vi "main.vi"() -> ()   [LabVIEW 2018]
uses:
  <vilib>/Utility/config.llb/Write Key (Double).vi
  <vilib>/Utility/config.llb/Write Key (U32).vi
  <vilib>/Utility/config.llb/Write Key (Boolean).vi
  <vilib>/Utility/config.llb/Write Key (I32).vi
  <vilib>/Utility/config.llb/NI_LVConfig.lvlib
panel:
  in  "脉冲开关 2":bool
  in  "选项卡控件":enum32{"Graph", "All channel", "Single channel"}(tab)
  out "波形图表时间簇1":cluster{"起始":dbl, "中间":dbl, "终止":dbl}={"起始"=0.0, "中间"=2.5, "终止"=5.0} {"起始" format="%#.1p"; "终止" format="%#.1p"; "中间" format="%#.1p"}
  out "Chart1":waveform(dbl)[](graph)
  out "波形图表时间簇2":cluster{"起始":dbl, "中间":dbl, "终止":dbl}={"起始"=0.0, "中间"=2.5, "终止"=5.0} {"起始" format="%#.1p"; "终止" format="%#.1p"; "中间" format="%#.1p"}
  out "Chart2":waveform(dbl)[](graph)
  out "波形图表时间簇3":cluster{"起始":dbl, "中间":dbl, "终止":dbl}={"起始"=0.0, "中间"=2.5, "终止"=5.0} {"起始" format="%#.1p"; "终止" format="%#.1p"; "中间" format="%#.1p"}
  out "Chart3":waveform(dbl)[](graph)
  out "波形图表时间簇4":cluster{"起始":dbl, "中间":dbl, "终止":dbl}={"起始"=0.0, "中间"=2.5, "终止"=5.0} {"起始" format="%#.1p"; "终止" format="%#.1p"; "中间" format="%#.1p"}
  out "Chart4":waveform(dbl)[](graph)
  in  "全部":T1={"Amp"=1.0, "Fre"=2, "Wid"=20, "选通"=TRUE, "脉宽单位"=enum."us", "字符串"="全部", "Time"=2} {"Wid" min=1 step=1; "Amp" min=0 max=15 step=0.1 format="%#_3f"}
  in  "所有保存配置":bool
  out "Path":path
  in  "单独保存配置":bool
  in  "读取配置":bool
  in  "Configuration select":path
  out "Configuration save":path
  in  "Information":T2(array[cluster])=[[{"Amp"=10.0, "Fre"=1, "Wid"=200, "选通"=TRUE, "脉宽单位"=enum."us", "字符串"="CH0", "Time"=1}, {"Amp"=2.0, "Fre"=2, "Wid"=200, "选通"=FALSE, "脉宽单位"=enum."us", "字符串"="CH1", "Time"=2}, {"Amp"=1.0, "Fre"=3, "Wid"=200, "选通"=FALSE, "脉宽单位"=enum."us", "字符串"="CH2", "Time"=3}, {"Amp"=1.0, "Fre"=4, "Wid"=200, "选通"=FALSE, "脉宽单位"=enum."us", "字符串"="CH3", "Time"=4}, {"Amp"=2.0, "Fre"=5, "Wid"=200, "选通"=FALSE, "脉宽单位"=enum."us", "字符串"="CH4", "Time"=5}, {"Amp"=3.0, "Fre"=6, "Wid"=200, "选通"=FALSE, "脉宽单位"=enum."us", "字符串"="CH5", "Time"=6}, {"Amp"=2.0, "Fre"=7, "Wid"=200, "选通"=FALSE, "脉宽单位"=enum."us", "字符串"="CH6", "Time"=7}, {"Amp"=10.0, "Fre"=8, "Wid"=200, "选通"=FALSE, "脉宽单位"=enum."us", "字符串"="CH7", "Time"=8}], [{"Amp"=1.0, "Fre"=1, "Wid"=200, "选通"=FALSE, "脉宽单位"=enum."us", "字符串"="CH8", "Time"=9}, {"Amp"=1.0, "Fre"=2, "Wid"=200, "选通"=FALSE, "脉宽单位"=enum."us", "字符串"="CH9", "Time"=10}, {"Amp"=1.0, "Fre"=3, "Wid"=200, "选通"=FALSE, "脉宽单位"=enum."us", "字符串"="CH10", "Time"=11}, {"Amp"=1.0, "Fre"=4, "Wid"=200, "选通"=FALSE, "脉宽单位"=enum."us", "字符串"="CH11", "Time"=12}, {"Amp"=1.0, "Fre"=5, "Wid"=200, "选通"=TRUE, "脉宽单位"=enum."us", "字符串"="CH12", "Time"=13}, {"Amp"=1.0, "Fre"=6, "Wid"=200, "选通"=FALSE, "脉宽单位"=enum."us", "字符串"="CH13", "Time"=14}, {"Amp"=1.0, "Fre"=7, "Wid"=200, "选通"=FALSE, "脉宽单位"=enum."us", "字符串"="CH14", "Time"=15}, {"Amp"=1.0, "Fre"=8, "Wid"=200, "选通"=FALSE, "脉宽单位"=enum."us", "字符串"="CH15", "Time"=16}], [{"Amp"=1.0, "Fre"=1, "Wid"=200, "选通"=FALSE, "脉宽单位"=enum."us", "字符串"="CH16", "Time"=1}, {"Amp"=1.0, "Fre"=2, "Wid"=200, "选通"=FALSE, "脉宽单位"=enum."us", "字符串"="CH17", "Time"=2}, {"Amp"=1.0, "Fre"=3, "Wid"=200, "选通"=FALSE, "脉宽单位"=enum."us", "字符串"="CH18", "Time"=3}, {"Amp"=1.0, "Fre"=4, "Wid"=200, "选通"=TRUE, "脉宽单位"=enum."us", "字符串"="CH19", "Time"=4}, {"Amp"=1.0, "Fre"=5, "Wid"=200, "选通"=FALSE, "脉宽单位"=enum."us", "字符串"="CH20", "Time"=5}, {"Amp"=1.0, "Fre"=6, "Wid"=200, "选通"=TRUE, "脉宽单位"=enum."us", "字符串"="CH21", "Time"=6}, {"Amp"=1.0, "Fre"=7, "Wid"=200, "选通"=FALSE, "脉宽单位"=enum."us", "字符串"="CH22", "Time"=7}, {"Amp"=1.0, "Fre"=8, "Wid"=200, "选通"=FALSE, "脉宽单位"=enum."us", "字符串"="CH23", "Time"=8}], [{"Amp"=1.0, "Fre"=1, "Wid"=200, "选通"=FALSE, "脉宽单位"=enum."us", "字符串"="CH24", "Time"=1}, {"Amp"=1.0, "Fre"=2, "Wid"=200, "选通"=FALSE, "脉宽单位"=enum."us", "字符串"="CH25", "Time"=2}, {"Amp"=1.0, "Fre"=2, "Wid"=200, "选通"=FALSE, "脉宽单位"=enum."us", "字符串"="CH26", "Time"=3}, {"Amp"=1.0, "Fre"=2, "Wid"=200, "选通"=FALSE, "脉宽单位"=enum."us", "字符串"="CH27", "Time"=4}, {"Amp"=1.0, "Fre"=2, "Wid"=200, "选通"=FALSE, "脉宽单位"=enum."us", "字符串"="CH28", "Time"=5}, {"Amp"=1.0, "Fre"=31, "Wid"=200, "选通"=FALSE, "脉宽单位"=enum."us", "字符串"="CH29", "Time"=6}, {"Amp"=1.0, "Fre"=31, "Wid"=200, "选通"=FALSE, "脉宽单位"=enum."us", "字符串"="CH30", "Time"=7}, {"Amp"=1.0, "Fre"=31, "Wid"=200, "选通"=TRUE, "脉宽单位"=enum."us", "字符串"="CH31", "Time"=8}]] {"Wid" min=1 step=1; "Amp" min=0 max=15 step=0.1 format="%#_3f"}
  in  "Save path":path=path "C:/Users/86131/Desktop/新建文件夹"
  in  "打开TDMS":bool
  out "Record status":string
  in  "波形图表时间簇4 2":cluster{"起始":dbl, "中间":dbl, "终止":dbl} {"起始" format="%#.1p"; "终止" format="%#.1p"; "中间" format="%#.1p"}
  out "记录文件输出路径":path
  out "Countdown(s)":dbl format="%<%H:%M:%S>t"
  in  "Reocord mode":T3(ring)
  in  "Duration(s)":u32=10
  in  "Interval time(s)":i32=60 format="%<%H:%M:%S>t"
  in  "倒计时控制":bool
  out "tdms文件输出":refnum<k34>
  out "采集时间已到":bool
  in  "XScale":dbl(ring)=5.0 items=["10ms"=0.01, "100ms"=0.1, "1s"=1.0, "5s"=5.0, "10s"=10.0]
  in  "YScale":i16(ring)=5000 items=["+/-50μV"=50, "+/-100μV"=100, "+/-200μV"=200, "+/-500μV"=500, "+/-1mV"=1000, "+/-2mV"=2000, "+/-5mV"=5000, "+/-10mV"=10000]
  out "停止控制":bool=TRUE
  in  "停止按钮":bool
  in  "开始按钮":bool
  in  "记录开关":bool
  in  "脉冲开关":bool
  in  "命名方式":enum16{"电穿孔条件", "时间"}(ring)=enum."时间"
  # "Cell electrophysiological \nrecording system"
  # "Fixed time setting"
  # "CH0"
  # "CH1"
  # "CH2"
  # "CH3"
  # "CH4"
  # "CH5"
  # "CH6"
  # "CH7"
  # "CH8"
  # "CH9"
  # "CH10"
  # "CH11"
  # "CH12"
  # "CH13"
  # "CH14"
  # "CH15"
  # "CH16"
  # "CH17"
  # "CH18"
  # "CH19"
  # "CH20"
  # "CH21"
  # "CH22"
  # "CH23"
  # "CH24"
  # "CH25"
  # "CH26"
  # "CH27"
  # "CH28"
  # "CH29"
  # "CH30"
  # "CH31"
  # "V"
  # "Hz"
  # "s"
  # "V"
  # "Hz"
  # "s"
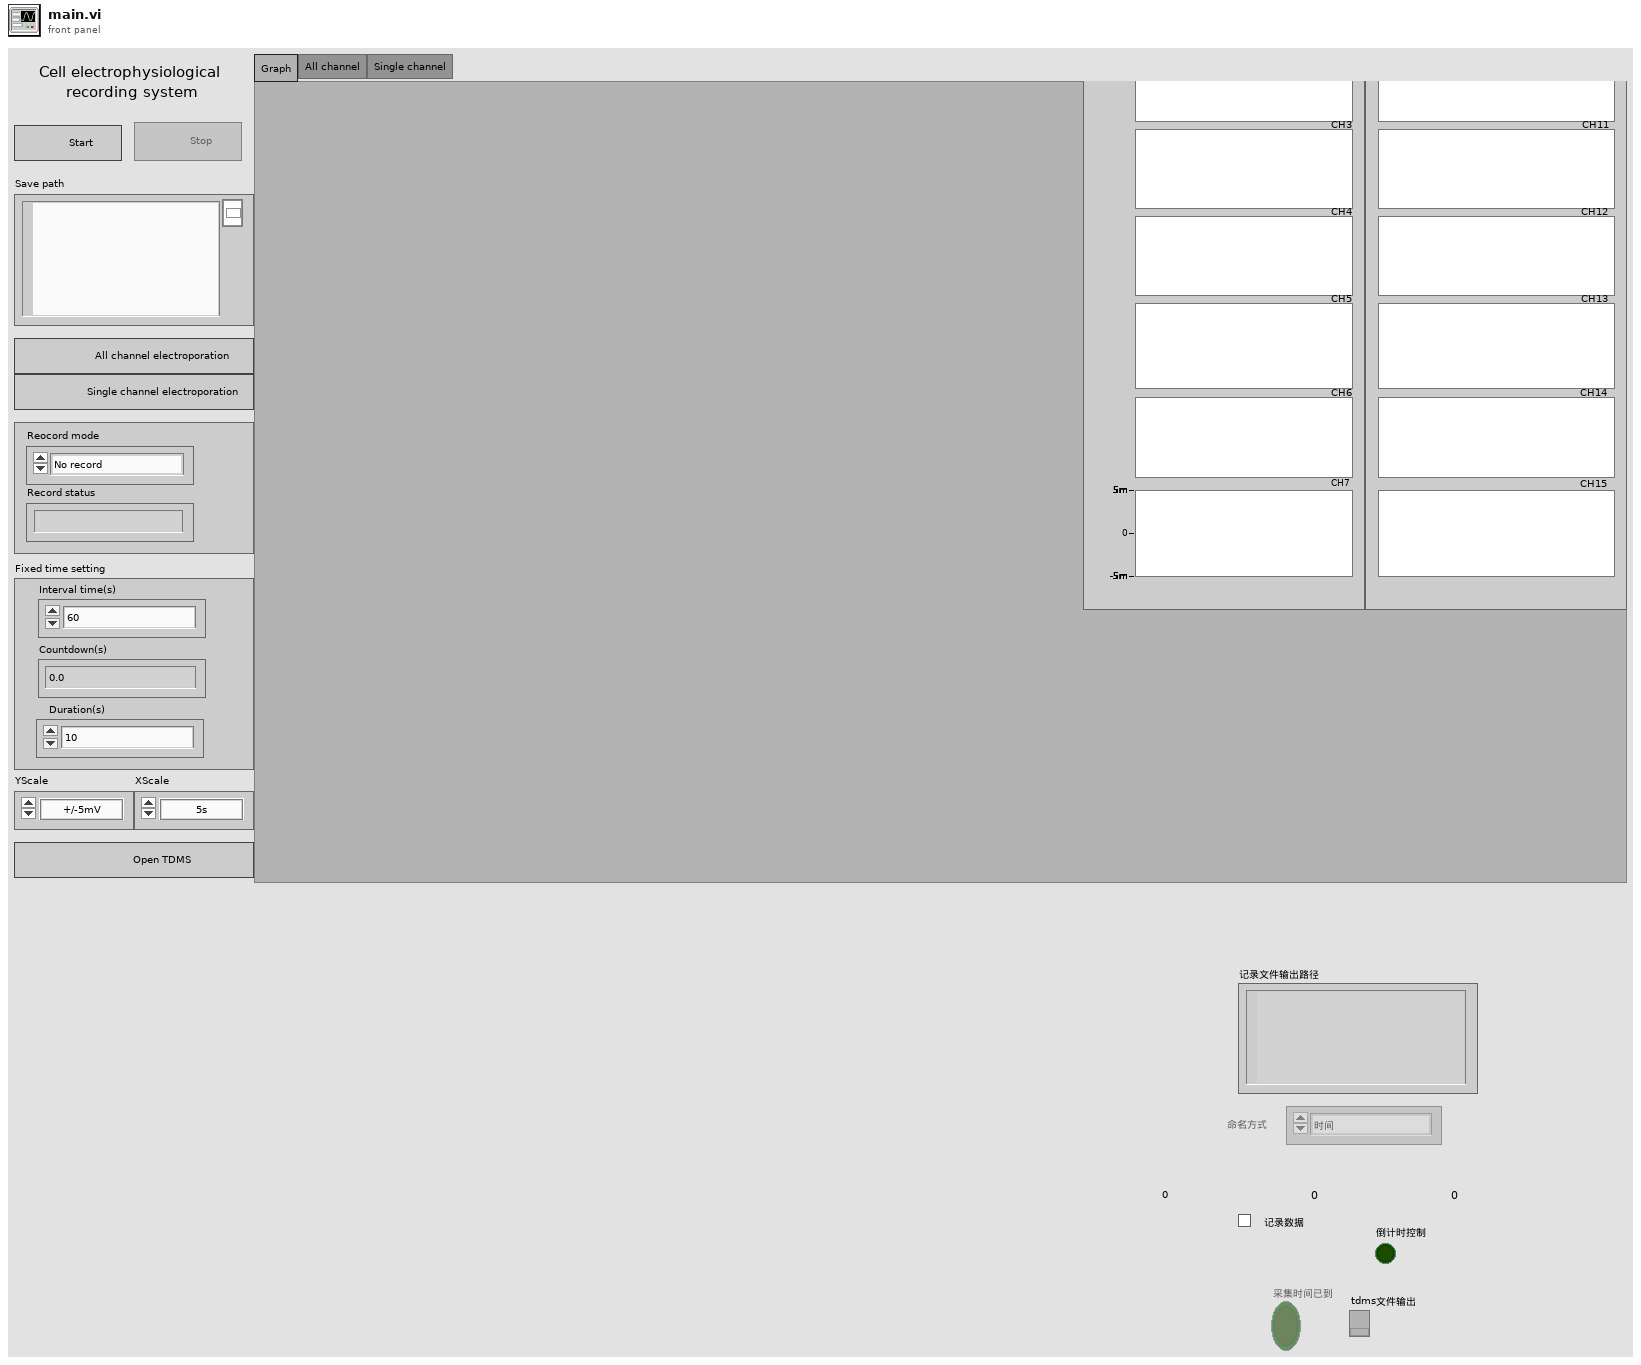
[diagram p1: front panel]
types:
  T1 = cluster{"Amp":sgl, "Fre":u32, "Wid":u16, "选通":bool, "脉宽单位":enum16{"ns", "us", "ms"}, "字符串":string, "Time":i32}
  T2 = cluster{"Amp":sgl, "Fre":u32, "Wid":u16, "选通":bool, "脉宽单位":enum16{"ns", "us", "ms"}, "字符串":string, "Time":i32}[][]
  T3 = enum16{"No record", "Continuous record", "Fixed time"}
  T4 = enum16{"open", "open or create", "create or replace", "create", "open (read-only)"}
  T5 = enum8{"Enabled", "Disabled", "Disabled and Grayed Out"}
  T6 = typedef "NI_LVConfig.lvlib/Config Data RefNum.ctl" = refnum<k1>
  T7 = cluster{"幅值":sgl, "频率":u32, "脉宽":u16, "选通":bool, "脉宽单位":enum16{"ns", "us", "ms"}, "字符串":string, "时间":i32}[][]
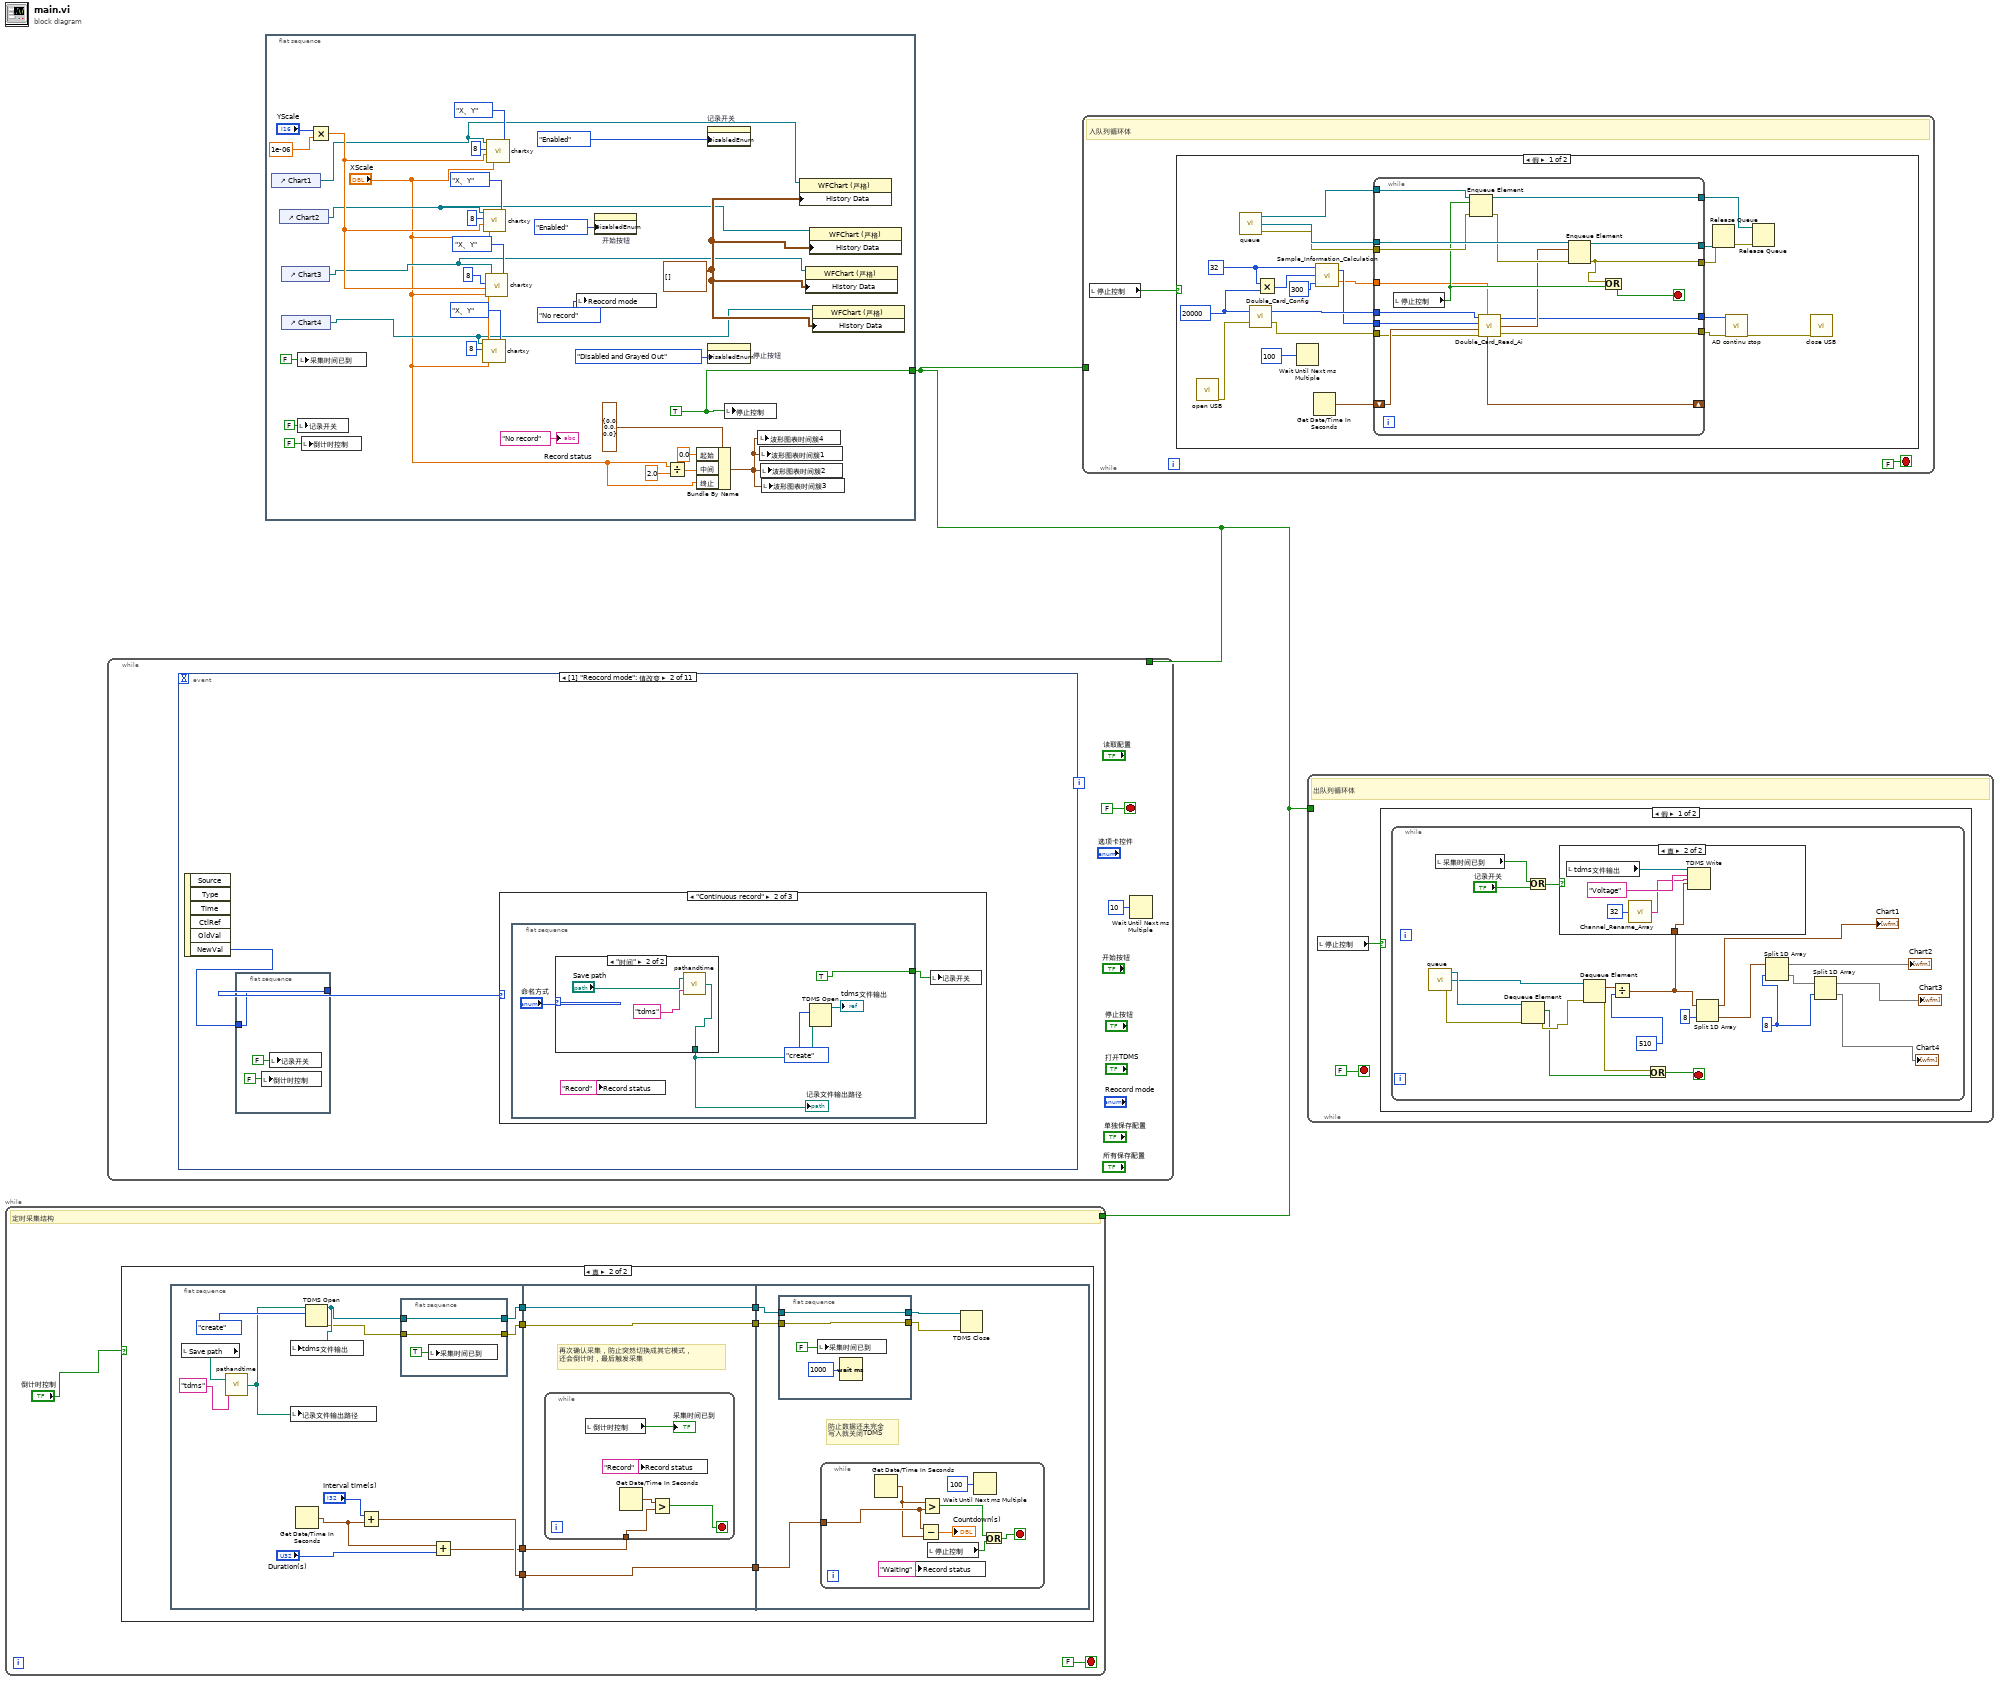
[diagram p0: block diagram]
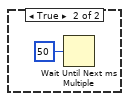
[diagram p3: hidden frame]
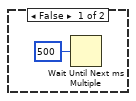
[diagram p4: hidden frame]
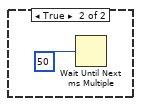
[diagram p5: hidden frame]
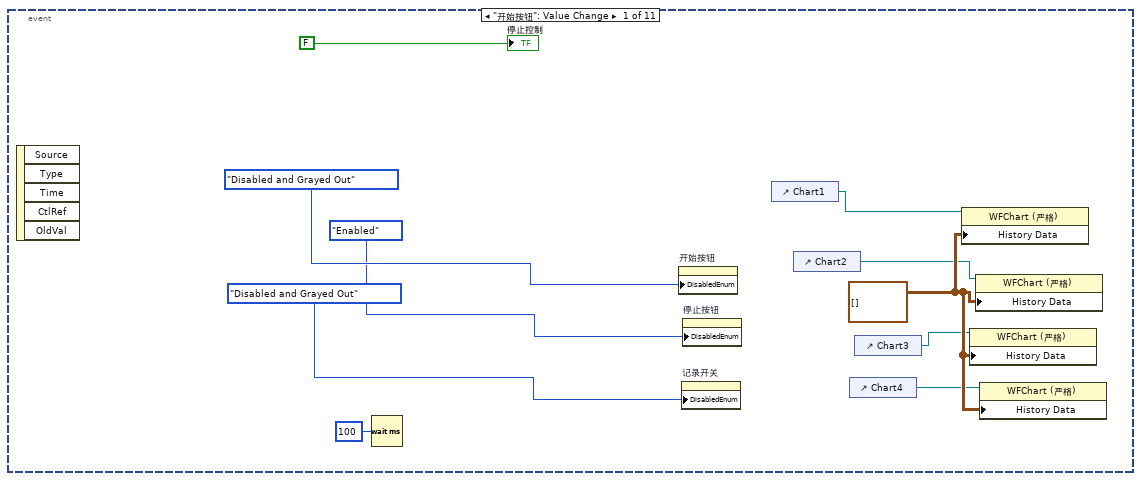
[diagram p6: hidden frame]
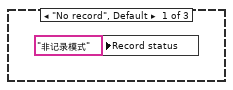
[diagram p7: hidden frame]
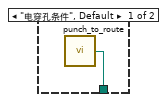
[diagram p8: hidden frame]
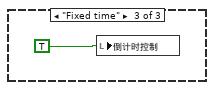
[diagram p9: hidden frame]
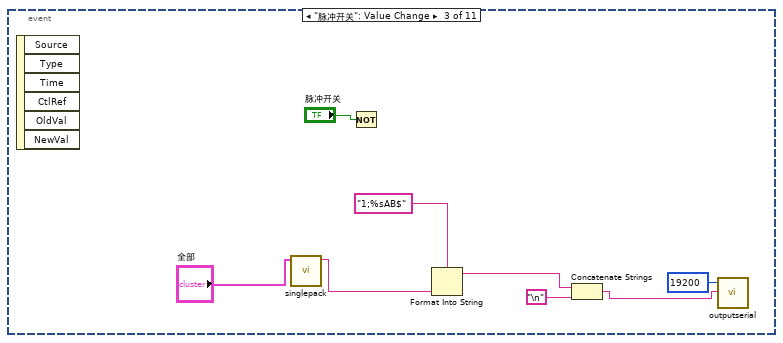
[diagram p10: hidden frame]
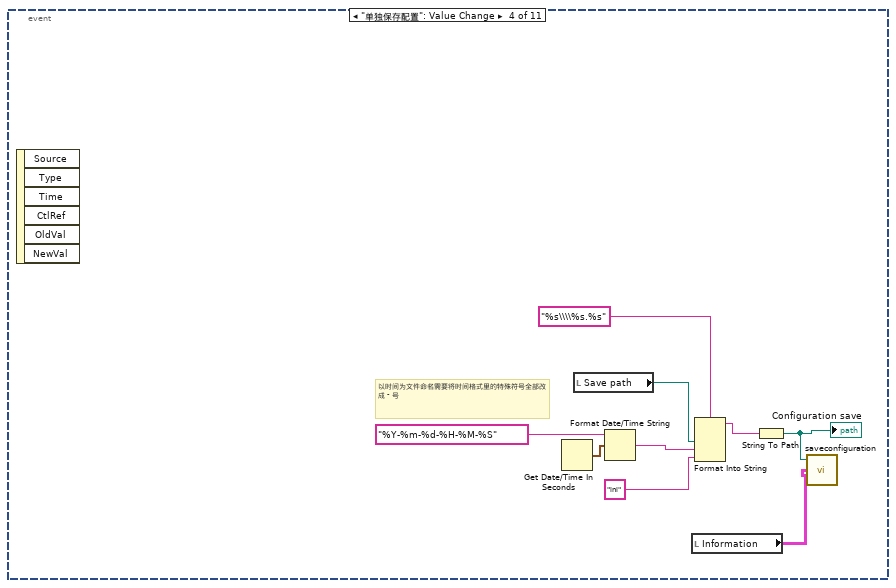
[diagram p11: hidden frame]
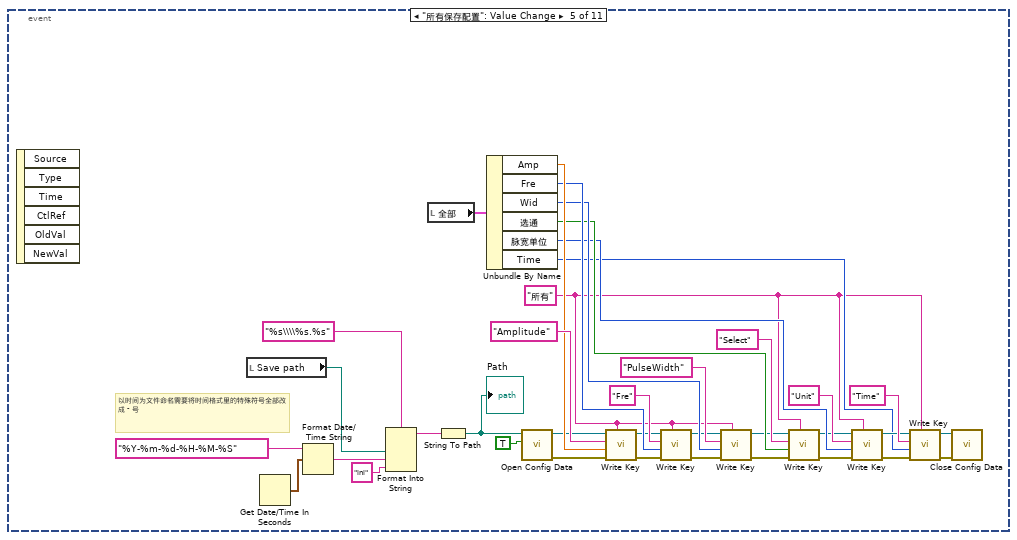
[diagram p12: hidden frame]
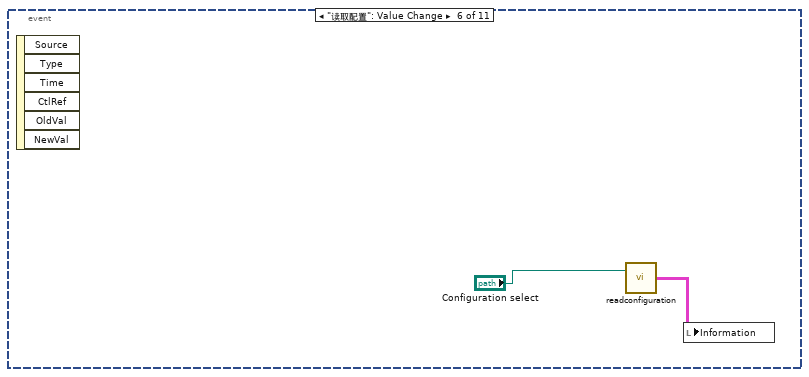
[diagram p13: hidden frame]
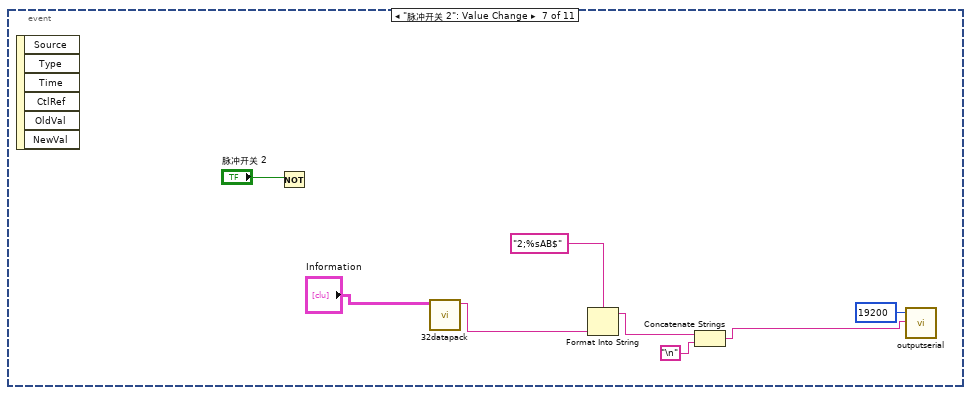
[diagram p14: hidden frame]
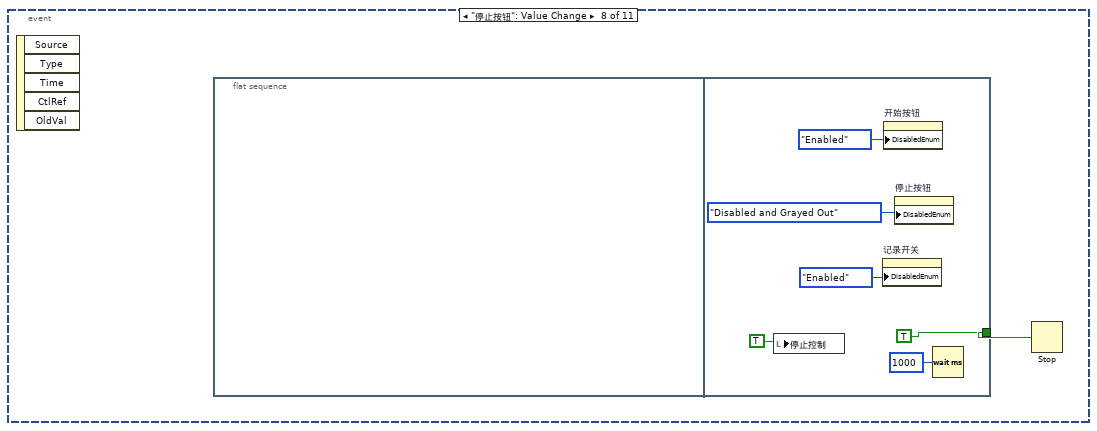
[diagram p15: hidden frame]
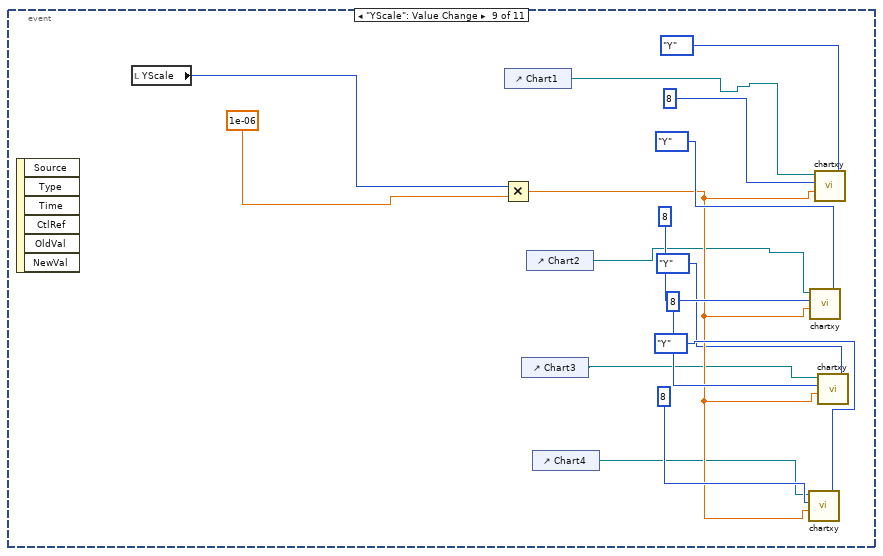
[diagram p16: hidden frame]
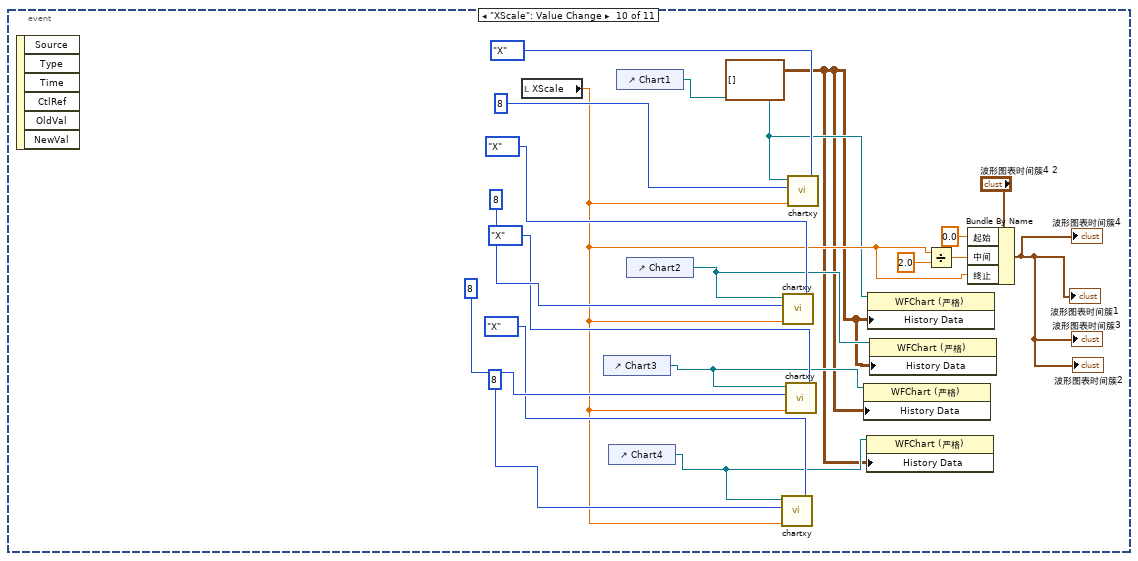
[diagram p17: hidden frame]
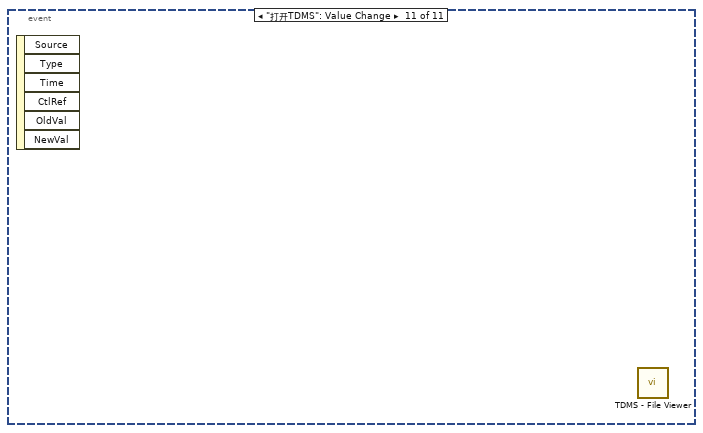
[diagram p18: hidden frame]
diagram:
  n1 = while {
    tunnel: w1 -> [_]
    stop <- FALSE stop-if-true
    # "定时采集结构"
    n2 = case shown="真" "倒计时控制" {
      frame False {
        n3 = Wait Until Next ms Multiple(millisecond multiple=u32 500 ("等待时间（毫秒）")) -> ()  [unwired: 1 out]
      }
      frame True {
        n4 = flat-sequence {
          tunnel: [w18] -> w11
          tunnel: [w16] -> w10
          tunnel: [w22] -> w6
          tunnel: [w19] -> w5
          tunnel: w11 -> [w31]
          tunnel: w10 -> [w30]
          tunnel: [w31] -> w9
          tunnel: [w30] -> w8
          tunnel: [w29] -> w7
          tunnel: w6 -> [w29]
          tunnel: w5 -> [w28]
          tunnel: w9 -> [w39]
          tunnel: w8 -> [w37]
          tunnel: w7 -> [w41]
          frame #0 {
            n5 = local read "Save path"() -> (w12:path)
            n6 = call "pathandtime.vi"("文件扩展名"="tdms", "文件路径输入控件"=w12) -> ("时间命名的文件路径"=w13:path)
            n7 = local write "记录文件输出路径"(w13) -> ()
            n8 = Get Date/Time In Seconds() -> (seconds since 1Jan1904=w20:timestamp)
            n9 = TDMS Open(10:T4."create" ("操作(0:open)"), 11:w13) -> (0:w15:errorcluster, 3:w17:refnum<k34>)  [unwired: 5 in]
            n10 = local write "tdms文件输出"(w17) -> ()
            n11 = Add(x="Interval time(s)", y=w20) -> (x+y=w22:timestamp)
            n12 = flat-sequence {
              tunnel: [w27] -> w18
              tunnel: w17 -> [w27]
              tunnel: [w26] -> w16
              tunnel: w15 -> [w26]
              frame #0 {
                n13 = local write "采集时间已到"(TRUE ("采集时间已到")) -> ()
              }
            }
            n14 = Add(x=w20, y="Duration(s)") -> (x+y=w19:timestamp)
          }
          frame #1 {
            # "再次确认采集，防止突然切换成其它模式，\n还会倒计时，最后触发采集"
            n15 = while {
              tunnel: w28 -> [w34]
              stop <- w33 stop-if-true
              n16 = local read "倒计时控制"() -> (→"采集时间已到":bool)
              n17 = Get Date/Time In Seconds() -> (seconds since 1Jan1904=w35:timestamp)
              n18 = local write "Record status"("Record" ("记录状态")) -> ()
              n19 = Greater?(x=w35, y=w34) -> (0:w33:bool)
            }
          }
          frame #2 {
            # "防止数据还未完全\n写入就关闭TDMS"
            n20 = flat-sequence {
              tunnel: [w44] -> w40
              tunnel: w39 -> [w44]
              tunnel: [w43] -> w38
              tunnel: w37 -> [w43]
              frame #0 {
                n21 = local write "采集时间已到"(FALSE ("布尔 2")) -> ()
                n22 = Wait (ms)(milliseconds to wait=u32 1000 ("毫秒倍数")) -> ()  [unwired: 1 out]
              }
            }
            n23 = while {
              tunnel: w41 -> [w52]
              stop <- w47 stop-if-true
              n24 = Get Date/Time In Seconds() -> (seconds since 1Jan1904=w51:timestamp)
              n25 = local write "Record status"("Waiting" ("记录状态")) -> ()
              n26 = Subtract(x=w52, y=w51) -> (x-y=→"Countdown(s)":dbl)
              n27 = Greater?(x=w51, y=w52) -> (0:w49:bool)
              n28 = local read "停止控制"() -> (w48:bool)
              n29 = Wait Until Next ms Multiple(millisecond multiple=u32 100 ("毫秒倍数")) -> ()  [unwired: 1 out]
              n30 = Or(x=w49, y=w48) -> (x .or. y?=w47:bool)
            }
            n31 = TDMS Close(8:w38, 11:w40) -> ()  [unwired: 2 out]
          }
        }
      }
    }
  }
  n32 = while {
    tunnel: w1 -> [_]
    stop <- FALSE stop-if-true
    n33 = event shown="[1] \"Reocord mode\": 值改变" {
      selector: _ -> [_ _ _ _ _ _ _ _ _ _ _]
      dyn-events: _ -> [_ _ _ _ _ _ _ _ _ _ _]
      timeout: _ -> [_ _ _ _ _ _ _ _ _ _ _]
      event "开始按钮": Value Change {
        w61 = waveform(dbl)[][] [] ("历史数据")
        n34 = event-data() -> ()  [unwired: 1 in, 5 out]
        n35 = Wait (ms)(milliseconds to wait=u32 100 ("毫秒倍数")) -> ()  [unwired: 1 out]
        n36 = property on="开始按钮" class="Bool"("DisabledEnum"=T5."Disabled and Grayed Out" ("禁用")) -> ()  [unwired: 2 in, 2 out]
        n37 = property on="记录开关" class="Bool (严格)"("DisabledEnum"=T5."Disabled and Grayed Out" ("禁用")) -> ()  [unwired: 2 in, 2 out]
        n38 = property on="停止按钮" class="Bool"("DisabledEnum"=T5."Enabled" ("禁用")) -> ()  [unwired: 2 in, 2 out]
        n39 = control-ref of="Chart1"() -> (w60:refnum<vi>)
        n40 = control-ref of="Chart2"() -> (w59:refnum<vi>)
        n41 = control-ref of="Chart4"() -> (w57:refnum<vi>)
        n42 = control-ref of="Chart3"() -> (w58:refnum<vi>)
        n43 = property on="属性节点" class="WFChart (严格)"(reference=w60, "History Data"=w61) -> ()  [unwired: 1 in, 2 out]
        n44 = property on="属性节点" class="WFChart (严格)"(reference=w58, "History Data"=w61) -> ()  [unwired: 1 in, 2 out]
        n45 = property on="属性节点" class="WFChart (严格)"(reference=w59, "History Data"=w61) -> ()  [unwired: 1 in, 2 out]
        n46 = property on="属性节点" class="WFChart (严格)"(reference=w57, "History Data"=w61) -> ()  [unwired: 1 in, 2 out]
        "停止控制" <- FALSE ("停止控制")
      }
      event "Reocord mode": Value Change {
        n47 = event-data() -> ("NewVal"=w66:T3)  [unwired: 1 in, 5 out]
        n48 = flat-sequence {
          tunnel: w66 -> [w70]
          tunnel: [w70] -> w67
          frame #0 {
            n49 = local write "倒计时控制"(FALSE ("倒计时控制")) -> ()
            n50 = local write "记录开关"(FALSE ("记录开关")) -> ()
          }
        }
        n51 = case shown="\"Continuous record\"" w67 {
          frame "No record", Default {
            n52 = local write "Record status"("非记录模式" ("记录状态")) -> ()
          }
          frame "Continuous record" {
            n53 = flat-sequence {
              tunnel: [TRUE ("记录开关")] -> w72
              frame #0 {
                n54 = case shown="\"时间\"" "命名方式" {
                  tunnel: [w79 w81] -> w74
                  frame "电穿孔条件", Default {
                    n55 = call "punch_to_route.vi"() -> ("电穿孔条件命名"=w79:path)  [unwired: 2 in]
                  }
                  frame "时间" {
                    n56 = call "pathandtime.vi"("文件扩展名"="tdms", "文件路径输入控件"="Save path") -> ("时间命名的文件路径"=w81:path)
                  }
                }
                "记录文件输出路径" <- w74
                n57 = local write "Record status"("Record" ("记录状态")) -> ()
                n58 = TDMS Open(10:T4."create" ("操作(0:open)"), 11:w74) -> (3:→"tdms文件输出":refnum<k34>)  [unwired: 5 in, 1 out]
              }
            }
            n59 = local write "记录开关"(w72) -> ()
          }
          frame "Fixed time" {
            n60 = local write "倒计时控制"(TRUE ("倒计时控制")) -> ()
          }
        }
      }
      event "脉冲开关": Value Change {
        n61 = event-data() -> ()  [unwired: 1 in, 6 out]
        n62 = call "singlepack.vi"("脉冲属性 2"="全部") -> ("字符串"=w88:string)  [unwired: 10 in]
        n63 = Not(x="脉冲开关") -> ()  [unwired: 1 out]
        n64 = Format Into String(format string="1;%sAB$" ("格式字符串"), w88) -> (resulting string=w86:string)  [unwired: 2 in, 1 out]
        n65 = Concatenate Strings(w86, "\n") -> (w85:string)
        n66 = call "outputserial.vi"("发送数据"=w85, "通讯波特率"=u32 19200) -> ()  [unwired: 1 in]
      }
      event "单独保存配置": Value Change {
        # "以时间为文件命名需要将时间格式里的特殊符号全部改成 - 号"
        n67 = event-data() -> ()  [unwired: 1 in, 6 out]
        n68 = Get Date/Time In Seconds() -> (seconds since 1Jan1904=w97:timestamp)
        n69 = local read "Save path"() -> (w92:path)
        n70 = Format Date/Time String(time format string (%c)="%Y-%m-%d-%H-%M-%S" ("时间格式字符串(%c)"), seconds (now)=w97) -> (date/time string=w98:string)  [unwired: 1 in]
        n71 = local read "Information"() -> (w93:T2)
        n72 = Format Into String(format string="%s\\\\%s.%s" ("格式字符串"), w92, w98, "ini" ("输入 3")) -> (resulting string=w99:string)  [unwired: 2 in, 1 out]
        n73 = String To Path(string=w99) -> (path=w100:path)
        "Configuration save" <- w100
        n74 = call "saveconfiguration.vi"("脉冲信息"=w93, "配置文件的路径"=w100) -> ()  [unwired: 1 in]
      }
      event "所有保存配置": Value Change {
        w108 = "所有" ("格式字符串")
        # "以时间为文件命名需要将时间格式里的特殊符号全部改成 - 号"
        n75 = event-data() -> ()  [unwired: 1 in, 6 out]
        n76 = local read "Save path"() -> (w131:path)
        n77 = Get Date/Time In Seconds() -> (seconds since 1Jan1904=w135:timestamp)
        n78 = Format Date/Time String(time format string (%c)="%Y-%m-%d-%H-%M-%S" ("时间格式字符串(%c)"), seconds (now)=w135) -> (date/time string=w136:string)  [unwired: 1 in]
        n79 = Format Into String(format string="%s\\\\%s.%s" ("格式字符串"), w131, w136, "ini" ("输入 3")) -> (resulting string=w137:string)  [unwired: 2 in, 1 out]
        n80 = local read "全部"() -> (w103:T1)
        n81 = String To Path(string=w137) -> (path=w104:path)
        "Path" <- w104
        n82 = Unbundle By Name(w103) -> ("Amp"=w129:sgl, "Fre"=w124:u32, "Wid"=w123:u16, "选通"=w122:bool, "脉宽单位"=w121:enum16{"ns", "us", "ms"}, "Time"=w109:i32)
        n83 = call <vilib>:"Open Config Data.vi"("create file if necessary (T)"=TRUE, "configuration file path"=w104) -> ("error out"=w105:errorcluster, "refnum"=w106:T6)  [unwired: 7 in, 1 out]
        n84 = call-poly <vilib>:"Write Key.vi"("section"=w108, "error in (no error)"=w105, "value"=w129, "key"="Amplitude", "refnum"=w106) -> ("error out"=w116:errorcluster, "refnum out"=w120:T6)  [unwired: 4 in, 1 out]
        n85 = call-poly <vilib>:"Write Key.vi"("section"=w108, "error in (no error)"=w116, "value"=w124, "key"="Fre", "refnum"=w120) -> ("error out"=w115:errorcluster, "refnum out"=w119:T6)  [unwired: 4 in, 1 out]
        n86 = call-poly <vilib>:"Write Key.vi"("section"=w108, "error in (no error)"=w115, "value"=w123, "key"="PulseWidth", "refnum"=w119) -> ("error out"=w114:errorcluster, "refnum out"=w118:T6)  [unwired: 4 in, 1 out]
        n87 = call-poly <vilib>:"Write Key.vi"("section"=w108, "error in (no error)"=w114, "value"=w122, "key"="Select", "refnum"=w118) -> ("error out"=w113:errorcluster, "refnum out"=w117:T6)  [unwired: 4 in, 1 out]
        n88 = call-poly <vilib>:"Write Key.vi"("section"=w108, "error in (no error)"=w113, "value"=w121, "key"="Unit", "refnum"=w117) -> ("error out"=w110:errorcluster, "refnum out"=w111:T6)  [unwired: 4 in, 1 out]
        n89 = call-poly <vilib>:"Write Key.vi"("section"=w108, "error in (no error)"=w110, "value"=w109, "key"="Time", "refnum"=w111) -> ("error out"=w101:errorcluster, "refnum out"=w102:T6)  [unwired: 4 in, 1 out]
        n90 = call <vilib>:"Close Config Data.vi"("error in (no error)"=w101, "refnum"=w102) -> ()  [unwired: 8 in, 2 out]
      }
      event "读取配置": Value Change {
        n91 = event-data() -> ()  [unwired: 1 in, 6 out]
        n92 = call "readconfiguration.vi"("配置文件的路径"="Configuration select") -> ("脉冲信息"=w138:T7)  [unwired: 1 in]
        n93 = local write "Information"(w138) -> ()
      }
      event "脉冲开关 2": Value Change {
        n94 = event-data() -> ()  [unwired: 1 in, 6 out]
        n95 = Not(x="脉冲开关 2") -> ()  [unwired: 1 out]
        n96 = call "32datapack.vi"("脉冲信息"="Information") -> ("字符串"=w145:string)  [unwired: 10 in]
        n97 = Format Into String(format string="2;%sAB$" ("格式字符串"), w145) -> (resulting string=w143:string)  [unwired: 2 in, 1 out]
        n98 = Concatenate Strings(w143, "\n") -> (w141:string)
        n99 = call "outputserial.vi"("发送数据"=w141, "通讯波特率"=u32 19200) -> ()  [unwired: 1 in]
      }
      event "停止按钮": Value Change {
        n100 = event-data() -> ()  [unwired: 1 in, 5 out]
        n101 = flat-sequence {
          tunnel: [TRUE ("停止？(T)")] -> w148
          frame #0 {
          }
          frame #1 {
            n102 = local write "停止控制"(TRUE ("停止控制")) -> ()
            n103 = property on="记录开关" class="Bool (严格)"("DisabledEnum"=T5."Enabled" ("禁用")) -> ()  [unwired: 2 in, 2 out]
            n104 = property on="开始按钮" class="Bool"("DisabledEnum"=T5."Enabled" ("禁用")) -> ()  [unwired: 2 in, 2 out]
            n105 = property on="停止按钮" class="Bool"("DisabledEnum"=T5."Disabled and Grayed Out" ("禁用")) -> ()  [unwired: 2 in, 2 out]
            n106 = Wait (ms)(milliseconds to wait=u32 1000 ("等待时间（毫秒）")) -> ()  [unwired: 1 out]
          }
        }
        n107 = Stop(stop? (T)=w148) -> ()
      }
      event "YScale": Value Change {
        n108 = event-data() -> ()  [unwired: 1 in, 6 out]
        n109 = local read "YScale"() -> (w163:i16)
        n110 = Multiply(x=w163, y=1e-06) -> (x*y=w160:dbl)
        n111 = control-ref of="Chart1"() -> (w158:refnum<vi>)
        n112 = control-ref of="Chart3"() -> (w156:refnum<vi>)
        n113 = control-ref of="Chart2"() -> (w157:refnum<vi>)
        n114 = control-ref of="Chart4"() -> (w155:refnum<vi>)
        n115 = call "chartxy.vi"("选择调整的轴"=enum16{"Y", "X", "X、Y"}."Y", "Y标尺.最大值"=w160, "曲线数量"=u8 8, "波形图表引用输入"=w155) -> ()  [unwired: 1 in]
        n116 = call "chartxy.vi"("选择调整的轴"=enum16{"Y", "X", "X、Y"}."Y", "Y标尺.最大值"=w160, "曲线数量"=u8 8, "波形图表引用输入"=w157) -> ()  [unwired: 1 in]
        n117 = call "chartxy.vi"("选择调整的轴"=enum16{"Y", "X", "X、Y"}."Y", "Y标尺.最大值"=w160, "曲线数量"=u8 8, "波形图表引用输入"=w158) -> ()  [unwired: 1 in]
        n118 = call "chartxy.vi"("选择调整的轴"=enum16{"Y", "X", "X、Y"}."Y", "Y标尺.最大值"=w160, "曲线数量"=u8 8, "波形图表引用输入"=w156) -> ()  [unwired: 1 in]
      }
      event "XScale": Value Change {
        w170 = waveform(dbl)[][] [] ("历史数据")
        n119 = event-data() -> ()  [unwired: 1 in, 6 out]
        n120 = local read "XScale"() -> (w176:dbl)
        n121 = control-ref of="Chart3"() -> (w172:refnum<vi>)
        n122 = control-ref of="Chart4"() -> (w171:refnum<vi>)
        n123 = control-ref of="Chart1"() -> (w174:refnum<vi>)
        n124 = control-ref of="Chart2"() -> (w173:refnum<vi>)
        n125 = call "chartxy.vi"("选择调整的轴"=enum16{"Y", "X", "X、Y"}."X", "X标尺.长度"=w176, "曲线数量"=u8 8, "波形图表引用输入"=w171) -> ()  [unwired: 1 in]
        n126 = call "chartxy.vi"("选择调整的轴"=enum16{"Y", "X", "X、Y"}."X", "X标尺.长度"=w176, "曲线数量"=u8 8, "波形图表引用输入"=w173) -> ()  [unwired: 1 in]
        n127 = call "chartxy.vi"("选择调整的轴"=enum16{"Y", "X", "X、Y"}."X", "X标尺.长度"=w176, "曲线数量"=u8 8, "波形图表引用输入"=w172) -> ()  [unwired: 1 in]
        n128 = call "chartxy.vi"("选择调整的轴"=enum16{"Y", "X", "X、Y"}."X", "X标尺.长度"=w176, "曲线数量"=u8 8, "波形图表引用输入"=w174) -> ()  [unwired: 1 in]
        n129 = property on="属性节点" class="WFChart (严格)"(reference=w172, "History Data"=w170) -> ()  [unwired: 1 in, 2 out]
        n130 = property on="属性节点" class="WFChart (严格)"(reference=w171, "History Data"=w170) -> ()  [unwired: 1 in, 2 out]
        n131 = property on="属性节点" class="WFChart (严格)"(reference=w174, "History Data"=w170) -> ()  [unwired: 1 in, 2 out]
        n132 = property on="属性节点" class="WFChart (严格)"(reference=w173, "History Data"=w170) -> ()  [unwired: 1 in, 2 out]
        n133 = Divide(x=w176, y=2.0) -> (x/y=w177:dbl)
        n134 = Bundle By Name(cluster="波形图表时间簇4 2", "起始"=0.0, "中间"=w177, "终止"=w176) -> (→"波形图表时间簇2" →"波形图表时间簇3" →"波形图表时间簇4" →"波形图表时间簇1":cluster{"起始":dbl, "中间":dbl, "终止":dbl})
      }
      event "打开TDMS": Value Change {
        n135 = event-data() -> ()  [unwired: 1 in, 6 out]
        n136 = call <vilib>:"TDMS - File Viewer.vi"() -> ()  [unwired: 6 in, 2 out]
      }
    }
    n137 = Wait Until Next ms Multiple(millisecond multiple=u32 10 ("等待时间（毫秒）")) -> ()  [unwired: 1 out]
  }
  n138 = flat-sequence {
    tunnel: [w208] -> w1
    frame #0 {
      w208 = TRUE ("停止控制")
      w201 = waveform(dbl)[][] [] ("历史数据")
      n139 = control-ref of="Chart1"() -> (w200:refnum<vi>)
      n140 = control-ref of="Chart2"() -> (w199:refnum<vi>)
      n141 = control-ref of="Chart3"() -> (w198:refnum<vi>)
      n142 = control-ref of="Chart4"() -> (w197:refnum<vi>)
      n143 = local write "记录开关"(FALSE ("记录开关")) -> ()
      n144 = local write "采集时间已到"(FALSE ("采集时间已到")) -> ()
      n145 = local write "倒计时控制"(FALSE ("倒计时控制")) -> ()
      n146 = Multiply(x="YScale", y=1e-06) -> (x*y=w205:dbl)
      n147 = call "chartxy.vi"("选择调整的轴"=enum16{"Y", "X", "X、Y"}."X、Y", "X标尺.长度"="XScale", "Y标尺.最大值"=w205, "曲线数量"=u8 8, "波形图表引用输入"=w197) -> ()
      n148 = call "chartxy.vi"("选择调整的轴"=enum16{"Y", "X", "X、Y"}."X、Y", "X标尺.长度"="XScale", "Y标尺.最大值"=w205, "曲线数量"=u8 8, "波形图表引用输入"=w199) -> ()
      n149 = call "chartxy.vi"("选择调整的轴"=enum16{"Y", "X", "X、Y"}."X、Y", "X标尺.长度"="XScale", "Y标尺.最大值"=w205, "曲线数量"=u8 8, "波形图表引用输入"=w198) -> ()
      n150 = call "chartxy.vi"("选择调整的轴"=enum16{"Y", "X", "X、Y"}."X、Y", "X标尺.长度"="XScale", "Y标尺.最大值"=w205, "曲线数量"=u8 8, "波形图表引用输入"=w200) -> ()
      n151 = local write "Reocord mode"(T3."No record" ("Reocord mode")) -> ()
      n152 = property on="开始按钮" class="Bool"("DisabledEnum"=T5."Enabled" ("禁用")) -> ()  [unwired: 2 in, 2 out]
      n153 = Divide(x="XScale", y=2.0) -> (x/y=w193:dbl)
      n154 = Bundle By Name(cluster=cluster{"起始":dbl, "中间":dbl, "终止":dbl} {"起始"=0.0, "中间"=0.0, "终止"=0.0} ("波形图表时间簇4 2"), "起始"=0.0, "中间"=w193, "终止"="XScale") -> (w190:cluster{"起始":dbl, "中间":dbl, "终止":dbl})
      n155 = property on="记录开关" class="Bool (严格)"("DisabledEnum"=T5."Enabled" ("禁用")) -> ()  [unwired: 2 in, 2 out]
      n156 = property on="停止按钮" class="Bool"("DisabledEnum"=T5."Disabled and Grayed Out" ("禁用")) -> ()  [unwired: 2 in, 2 out]
      n157 = local write "停止控制"(w208) -> ()
      n158 = local write "波形图表时间簇4"(w190) -> ()
      n159 = local write "波形图表时间簇1"(w190) -> ()
      n160 = local write "波形图表时间簇2"(w190) -> ()
      n161 = local write "波形图表时间簇3"(w190) -> ()
      n162 = property on="属性节点" class="WFChart (严格)"(reference=w200, "History Data"=w201) -> ()  [unwired: 1 in, 2 out]
      n163 = property on="属性节点" class="WFChart (严格)"(reference=w198, "History Data"=w201) -> ()  [unwired: 1 in, 2 out]
      n164 = property on="属性节点" class="WFChart (严格)"(reference=w199, "History Data"=w201) -> ()  [unwired: 1 in, 2 out]
      n165 = property on="属性节点" class="WFChart (严格)"(reference=w197, "History Data"=w201) -> ()  [unwired: 1 in, 2 out]
      "Record status" <- "No record" ("记录状态")
    }
  }
  n166 = while {
    tunnel: w1 -> [_]
    stop <- FALSE stop-if-true
    # "入队列循环体"
    n167 = local read "停止控制"() -> (w220:bool)
    n168 = case shown="假" w220 {
      frame False {
        w230 = u8 32 ("通道数目")
        w229 = 20000 ("采样率(Hz)")
        n169 = call "open USB.vi"() -> ("error out"=w222:errorcluster)  [unwired: 10 in, 1 out]
        n170 = call "queue.vi"() -> ("控制队列输出"=w241:refnum<queue>, "数据队列输出"=w242:refnum<queue>, "错误输出"=w240:errorcluster)  [unwired: 2 in]
        n171 = call "Double_Card_Config.vi"("错误输入"=w222, "单通道采样率(Hz)"=w229) -> ("错误输出"=w233:errorcluster, "DevOut"=w234:i32)
        n172 = Multiply(x=w230, y=w229) -> (x*y=w228:i32)
        n173 = Wait Until Next ms Multiple(millisecond multiple=u32 100 ("等待时间（毫秒）")) -> ()  [unwired: 1 out]
        n174 = Get Date/Time In Seconds() -> (seconds since 1Jan1904=w232:timestamp)
        n175 = call "Sample_Information_Calculation.vi"("数据刷新周期(ms)"=u16 300, "总采样率(Hz)"=w228, "通道数目"=w230) -> ("单通道采样周期(s)"=w225:dbl, "采集点个数"=w226:u32)
        n176 = while {
          tunnel: w242 -> [w260]
          tunnel: w241 -> [w259]
          tunnel: w240 -> [w258]
          tunnel: [w257] -> w239
          tunnel: [w253] -> w238
          tunnel: [w255] -> w236
          tunnel: w234 -> [w246]
          tunnel: w233 -> [w245]
          shift-right: [w250] -> _
          shift-left: w232 -> [w251]
          tunnel: [w248] -> w224
          tunnel: [w247] -> w231
          tunnel: w226 -> [w244]
          tunnel: w225 -> [w243]
          stop <- w254 stop-if-true
          n177 = local read "停止控制"() -> (w252:bool)
          n178 = Enqueue Element(queue=w259, element=w252, error in (no error)=w258) -> (queue out=w255:refnum<queue>, error out=w256:errorcluster)  [unwired: 1 in, 1 out]
          n179 = call "Double_Card_Read_Ai.vi"("dev"=w246, "每通道采样周期(s)"=w243, "Points"=w244, "波形初始时间输入"=w251, "错误输入"=w245) -> ("波形初始时间输出"=w250:timestamp, "Dev out"=w248:i32, "数据输出"=w249:waveform(sgl)[], "error out"=w247:errorcluster)
          n180 = Enqueue Element(queue=w260, element=w249, error in (no error)=w256) -> (queue out=w257:refnum<queue>, error out=w253:errorcluster)  [unwired: 1 in, 1 out]
          n181 = Or(x=w253, y=w252) -> (x .or. y?=w254:bool)
        }
        n182 = Release Queue(queue=w239, error in (no error)=w238) -> (error out=w237:errorcluster)  [unwired: 1 in, 2 out]
        n183 = call "AD continu stop.vi"("error in (no error)"=w231, "dev"=w224) -> ("error out"=w223:errorcluster)  [unwired: 8 in, 1 out]
        n184 = Release Queue(queue=w236, error in (no error)=w237) -> ()  [unwired: 1 in, 3 out]
        n185 = call "close USB.vi"("error in (no error)"=w223) -> ()  [unwired: 9 in, 2 out]
      }
      frame True {
        n186 = Wait Until Next ms Multiple(millisecond multiple=u32 50 ("等待时间（毫秒）")) -> ()  [unwired: 1 out]
      }
    }
  }
  n187 = while {
    tunnel: w1 -> [_]
    stop <- FALSE stop-if-true
    # "出队列循环体"
    n188 = local read "停止控制"() -> (w262:bool)
    n189 = case shown="假" w262 {
      frame False {
        n190 = while {
          stop <- w284 stop-if-true
          w274 = 8 ("索引")
          n191 = call "queue.vi"() -> ("控制队列输出"=w271:refnum<queue>, "数据队列输出"=w270:refnum<queue>, "错误输出"=w269:errorcluster)  [unwired: 2 in]
          n192 = local read "采集时间已到"() -> (w276:bool)
          n193 = Dequeue Element(queue=w271, error in (no error)=w269) -> (element=w282:bool, error out=w283:errorcluster)  [unwired: 1 in, 2 out]
          n194 = Or(x=w276, y="记录开关") -> (x .or. y?=w278:bool)
          n195 = Dequeue Element(queue=w270, error in (no error)=w283) -> (element=w273:waveform(dbl)[], error out=w281:errorcluster)  [unwired: 1 in, 2 out]
          n196 = Divide(x=w273, y=510) -> (x/y=w268:waveform(dbl)[])
          n197 = case shown="真" w278 {
            tunnel: w268 -> [_ w289]
            frame False {
            }
            frame True {
              n198 = local read "tdms文件输出"() -> (w285:refnum<k34>)
              n199 = call "Channel_Rename_Array.vi"("通道数量"=u8 32) -> ("通道名称"=w286:string[])
              n200 = TDMS Write(0:w285, 5:"Voltage" ("组名称输入（无标题）"), 7:w286, 9:w289) -> ()  [unwired: 2 in, 4 out]
            }
          }
          n201 = Or(x=w281, y=w282) -> (x .or. y?=w284:bool)
          n202 = Split 1D Array(array=w268, index=8 ("索引")) -> (first subarray=→"Chart1":waveform(dbl)[], second subarray=w279:waveform(dbl)[])
          n203 = Split 1D Array(array=w279, index=w274) -> (first subarray=→"Chart2":waveform(dbl)[], second subarray=w275:waveform(dbl)[])
          n204 = Split 1D Array(array=w275, index=w274) -> (first subarray=→"Chart3":waveform(dbl)[], second subarray=→"Chart4":waveform(dbl)[])
        }
      }
      frame True {
        n205 = Wait Until Next ms Multiple(millisecond multiple=u32 50 ("等待时间（毫秒）")) -> ()  [unwired: 1 out]
      }
    }
  }
